vi "MMEM_STOR.vi"(0 "VISA IN":refnum<visa-resource-name>, 1 "File":string, 5 "error in":errorcluster, 7 "Type":string(combo)) -> (14 "VISA Out":refnum<visa-resource-name>, 19 "error out":errorcluster)   [LabVIEW 2018, in "PNA-X.lvlib"]
doc: "MMEMory:STORe[:<char>] <file> \n(Write-only) Stores the specified file (.sta, .cal, .csa, .cst, prn). \nTo save snp files, use Calc:Data:SNP:PORTs:SAVE. \nTo save *.cti files, use MMEM:STOR:CIT:DATA or MMEM:STOR:CIT:FORM. \nParameters \n<char> The type of file to store. Choose from: \nSTATe - Instrument states (.sta) \nCORRection - Calibration Data (.cal) \nCSARchive - Instrument state and calibration data (.csa) \nCSTate - Instrument state and link to Calibration data (.cst) \nNo <char> is specified for prn. \n1612\n\nIf <char> is unspecified, then the extension must be included in the filename. \nIf an extension is specified in <file> that does not agree with <char> then no \naction is taken. \nLearn about File Types \n<file> String - Name of any valid file that is not already in existence. See Specifying \nPath Names \nExamples MMEM:STOR:STAT 'myState' \nmmemory:store 'c:\\bin\\myState.sta' \nMMEM:STOR 'MyData.prn' \nQuery Syntax Not applicable \nDefault Not applicable"
uses:
  PNA-X.lvlib
panel:
  in  "Combo Box":string(combo)="CSA"
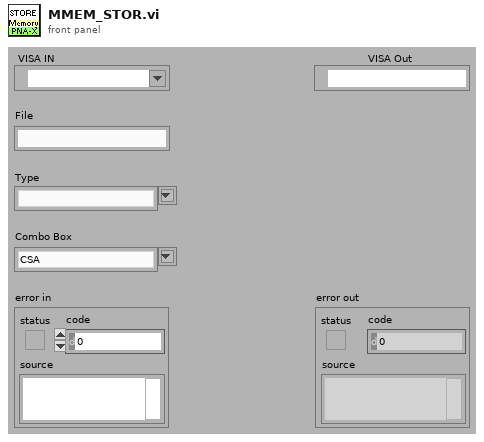
[diagram p1: front panel]
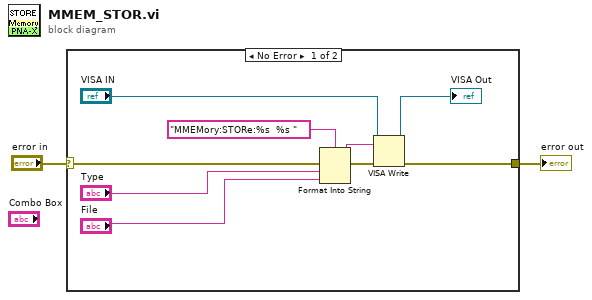
[diagram p0: block diagram]
diagram:
  n1 = case shown="No Error" "error in" {
    selector: "error in" -> [w11 w12]
    tunnel: [w6 w12] -> w1
    frame No Error {
      n2 = Format Into String(format string="MMEMory:STORe:%s  %s " ("Cmdline"), error in=w11, "Type", "File") -> (resulting string=w9:string, error out=w10:errorcluster)  [unwired: 1 in]
      n3 = VISA Write(VISA resource name="VISA IN", write buffer=w9, error in (no error)=w10) -> (VISA resource name out=→"VISA Out":refnum<visa-resource-name>, error out=w6:errorcluster)  [unwired: 1 out]
    }
    frame Error {
    }
  }
  "error out" <- w1
